vi "flattenToString.vi"(8 "error in (no error)":errorcluster, 10 "Record":refnum<class "Record.lvclass">, 11 "Serializer.JSON in":refnum<class "Serializer.JSON.lvclass">) -> (0 "error out":errorcluster, 2 "Flattened String":string, 3 "Serializer.JSON out":refnum<class "Serializer.JSON.lvclass">)   [LabVIEW 2017, in "Error Log.lvlib" / "Serializer.JSON.lvclass"]
uses:
  Serializer.JSON.lvclass
  Record/Record.lvclass
  <vilib>/LabVIEW Open Source Project/OpenSerializer JKI JSON/Serializer.JSON.lvclass
  C:/Program Files (x86)/National Instruments/LabVIEW 2017/vi.lib/LabVIEW Open Source Project/OpenSerializer/Serializer/Serializer.lvclass
  <vilib>/LabVIEW Open Source Project/OpenSerializer/Serializer/Serializer.lvclass
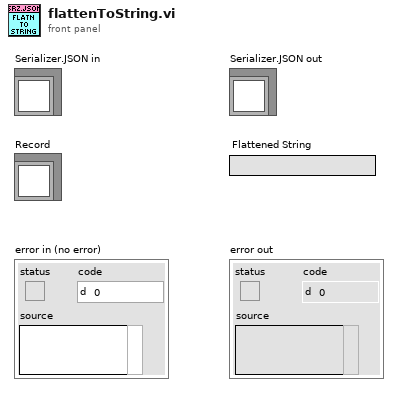
[diagram p1: front panel]
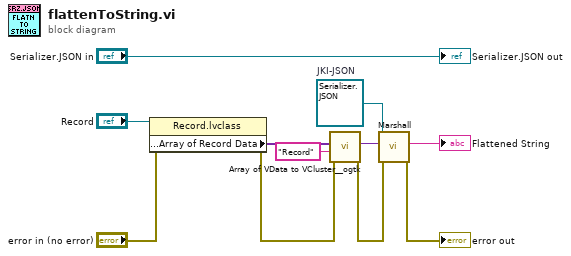
[diagram p0: block diagram]
diagram:
  w1 = refnum<class "Serializer.JSON.lvclass"> refnum  # JKI-JSON
  n1 = property class="Record.lvclass"(reference="Record", error in="error in (no error)") -> (error out=w6:errorcluster, "Public API:Properties:Array of Record Data"=w10:variant[])  [unwired: 1 out]
  n2 = call <userlib>:"Array of VData to VCluster__ogtk.vi"("error in (no error)"=w6, "Cluster Name"="Record", "Array"=w10) -> ("error out"=w4:errorcluster, "VCluster"=w5:variant)  [unwired: 7 in]
  n3 = call <vilib>:"Marshall.vi"("error in (no error)"=w4, "Variant"=w5, "Serializer in"=w1) -> ("error out"=→"error out":errorcluster, "String"=→"Flattened String":string)  [unwired: 6 in, 1 out]
  "Serializer.JSON out" <- "Serializer.JSON in"
